vi "Prototype.vi"(8 "error in (no error)":errorcluster, 10 "Target Method Prototyper in":refnum<class "Target Method Prototyper.lvclass">, 11 "Scripter in":refnum<class "Message Scripter.lvclass">) -> (0 "error out":errorcluster, 2 "Target Method Prototyper out":refnum<class "Target Method Prototyper.lvclass">, 3 "Scripter out":refnum<class "Message Scripter.lvclass">)   [LabVIEW 2020, in "Message Maker.lvlib" / "Target Method Prototyper.lvclass"]
uses:
  Target Method Prototyper.lvclass
  Message Maker.lvlib
  Message Scripter/Message Scripter.lvclass
  Prototyper/Prototyper.lvclass
  Target Method Icon Reader/Target Method Icon Reader.lvclass
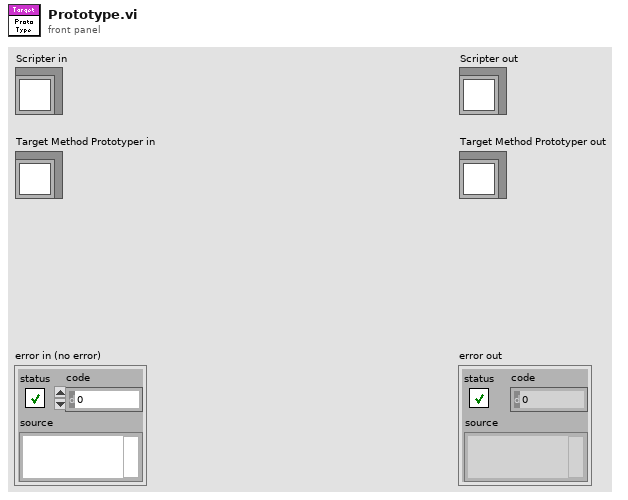
[diagram p1: front panel]
types:
  T1 = enum16{"Invalid Wire Rule", "Required", "Recommended", "Optional", "Dynamic Dispatch"}[]
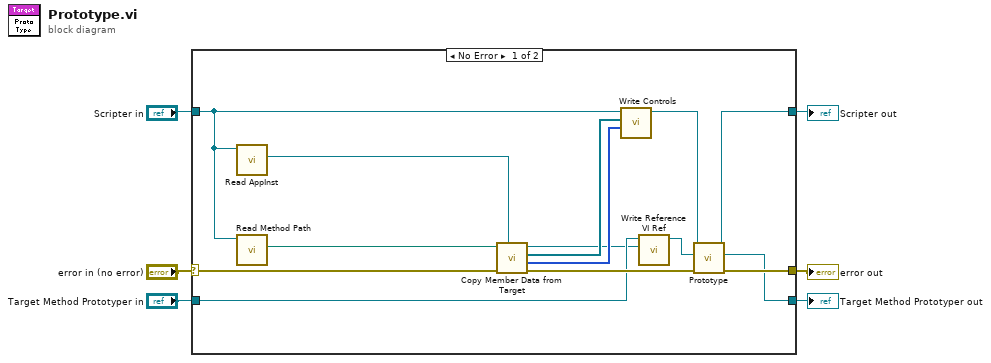
[diagram p0: block diagram]
diagram:
  n1 = case shown="No Error" "error in (no error)" {
    selector: "error in (no error)" -> [w20 w22]
    tunnel: "Scripter in" -> [w11 w23]
    tunnel: [w13 w23] -> w5
    tunnel: [w15 w22] -> w3
    tunnel: "Target Method Prototyper in" -> [w10 w21]
    tunnel: [w12 w21] -> w1
    frame No Error {
      n2 = call "Read AppInst.vi"("Message Maker in"=w11) -> ("AppInst"=w17:refnum<vi>)  [unwired: 10 in]
      n3 = call "Read Method Path.vi"("Message Maker in"=w11) -> ("Method Path"=w7:path)  [unwired: 10 in]
      n4 = call "Copy Member Data from Target.vi"("AppInst"=w17, "error in (no error)"=w20, "Target Method path"=w7) -> ("error out"=w16:errorcluster, "Wiring Rules"=w19:T1, "Controls[]"=w18:refnum<vi>[], "Target Method Ref"=w8:refnum<vi>)  [unwired: 5 in]
      n5 = call "Write Controls.vi"("Wiring Rules"=w19, "Controls[]"=w18, "Message Scripter in"=w11) -> ("Message Scripter out"=w14:refnum<class "Message Scripter.lvclass">)  [unwired: 8 in]
      n6 = call "Write Reference VI Ref.vi"("Reference VI Ref"=w8, "Prototyper in"=w10) -> ("Prototyper out"=w9:refnum<class "Target Method Prototyper.lvclass">)  [unwired: 9 in]
      n7 = call-parent "Prototype.vi"("error in (no error)"=w16, "Target Method Prototyper in"=w9, "Scripter in"=w14) -> ("error out"=w15:errorcluster, "Target Method Prototyper out"=w12:refnum<class "Target Method Prototyper.lvclass">, "Scripter out"=w13:refnum<class "Message Scripter.lvclass">)  [unwired: 6 in]
    }
    frame Error {
    }
  }
  "error out" <- w3
  "Target Method Prototyper out" <- w1
  "Scripter out" <- w5
